vi "Median with index.vi"(11 "Data in":dbl[](array[numeric])) -> (1 "Median Index":i32, 3 "Median Value":dbl)   [LabVIEW 2013]
uses:
  <vilib>/Analysis/NI_AALBase.lvlib
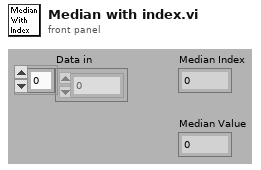
[diagram p1: front panel]
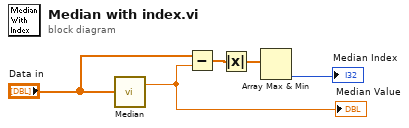
[diagram p0: block diagram]
diagram:
  n1 = call <vilib>:"Median.vi"("X"="Data in") -> ("median"=w1:dbl)  [unwired: 1 out]
  "Median Value" <- w1
  n2 = Subtract(x="Data in", y=w1) -> (x-y=w4:dbl[])
  n3 = Absolute Value(x=w4) -> (abs(x)=w3:dbl[])
  n4 = Array Max & Min(array=w3) -> (min index (indices)=→"Median Index":i32)  [unwired: 3 out]
